vi "integrate_imu.vi"(0 "fxp_imu_acc":fxp<+/-,32,16>, 5 "tape_detected":bool, 7 "fxp_tape_velocity":fxp<+/-,32,16>, 9 "fxp_tape_distance":u32, 11 "fxpe_imu_timestamp":fxp<+/-,64,32>) -> (6 "imu_velocity":fxp<+/-,32,16>, 10 "fxpe_imu_distance":fxp<+/-,64,32>)   [LabVIEW 2018]
uses:
  <vilib>/rvi/Emulation/niFpgaProcessEmulError.vi
  <vilib>/rvi/FXPMathLib/FxpAdd/XNode/nifxpmath_Add.xnode
  <vilib>/rvi/FXPMathLib/FxpMul/XNode/nifxpmath_Multiplier.xnode
  <vilib>/rvi/FXPMathLib/FxpSub/XNode/nifxpmath_Sub.xnode
  <vilib>/rvi/FXPMathLib/sim/FxpSim.dll
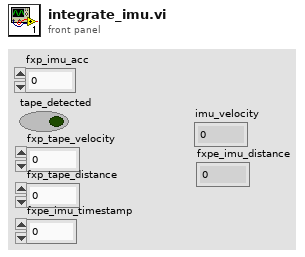
[diagram p1: front panel]
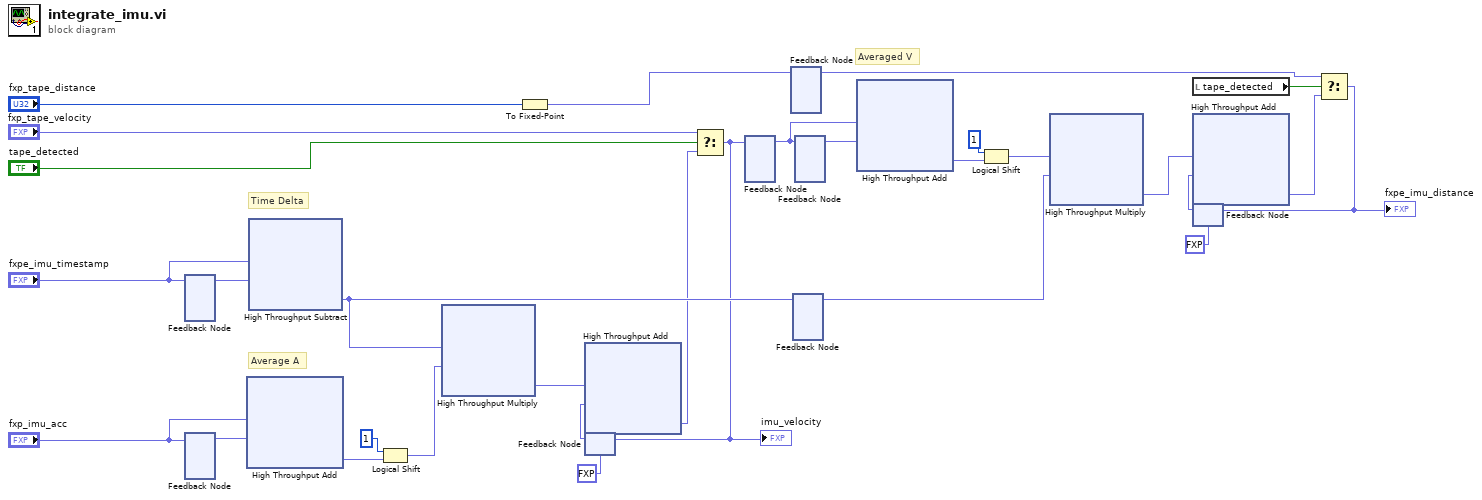
[diagram p0: block diagram]
diagram:
  # "Averaged V"
  # "Average A"
  # "Time Delta"
  n1 = feedback #1() -> (w5:fxp<+/-,64,32>)  [unwired: 1 in]
  n2 = feedback-in #1("fxpe_imu_timestamp") -> ()
  n3 = feedback #2() -> (w6:fxp<+/-,32,16>)  [unwired: 1 in]
  n4 = feedback-in #2("fxp_imu_acc") -> ()
  n5 = xnode ("High Throughput Add")("x"="fxp_imu_acc", "y"=w6) -> ("x+y"=w8:fxp<+/-,32,16>)
  n6 = xnode "High Throughput Subtract"("x"="fxpe_imu_timestamp", "y"=w5) -> ("x-y"=w28:fxp<+/-,64,32>)
  n7 = Logical Shift(y=i16 1, x=w8) -> (x << y=w10:fxp<+/-,32,16>)
  n8 = xnode ("High Throughput Multiply")("x"=w28, "y"=w10) -> ("x*y"=w13:fxp<+/-,48,16>)
  n9 = To Fixed-Point(number="fxp_tape_distance") -> (fixed-point=w30:fxp<+,32,32>)  [unwired: 1 in]
  n10 = feedback #3(fxp<+,1,1> 0.0) -> (w14:fxp<+/-,32,16>)
  n11 = xnode ("High Throughput Add")("x"=w13, "y"=w14) -> ("x+y"=w16:fxp<+/-,32,16>)
  n12 = Select(t="fxp_tape_velocity", s="tape_detected", f=w16) -> (s? t:f=w18:fxp<+/-,32,16>)
  "imu_velocity" <- w18
  n13 = feedback-in #3(w18) -> ()
  n14 = feedback-in #4(w18) -> ()
  n15 = feedback #4() -> (w3:fxp<+/-,32,16>)  [unwired: 1 in]
  n16 = feedback-in #5(w30) -> ()
  n17 = feedback #5() -> (w2:fxp<+,32,32>)  [unwired: 1 in]
  n18 = feedback-in #6(w28) -> ()
  n19 = feedback #6() -> (w1:fxp<+/-,64,32>)  [unwired: 1 in]
  n20 = feedback #7() -> (w17:fxp<+/-,32,16>)  [unwired: 1 in]
  n21 = feedback-in #7(w3) -> ()
  n22 = xnode ("High Throughput Add")("x"=w3, "y"=w17) -> ("x+y"=w20:fxp<+/-,32,16>)
  n23 = Logical Shift(y=i16 1, x=w20) -> (x << y=w27:fxp<+/-,32,16>)
  n24 = xnode ("High Throughput Multiply")("x"=w27, "y"=w1) -> ("x*y"=w29:fxp<+/-,48,16>)
  n25 = local read "tape_detected"() -> (w22:bool)
  n26 = feedback #8(fxp<+,1,1> 0.0) -> (w26:fxp<+/-,64,33>)
  n27 = xnode ("High Throughput Add")("x"=w29, "y"=w26) -> ("x+y"=w24:fxp<+/-,64,32>)
  n28 = Select(t=w2, s=w22, f=w24) -> (s? t:f=w25:fxp<+/-,64,33>)
  "fxpe_imu_distance" <- w25
  n29 = feedback-in #8(w25) -> ()
